vi "Autonomous Independent.vi"() -> ()   [LabVIEW 2016]
doc: "This VI is called when autonomous begins, and will automatically be terminated when autonomous ends. You can carry out timed or sensor driven robot movement independently without needing to return to the caller."
uses:
  Control Files/DriveMotors.ctl
  Control Files/SwerveMotors.ctl
panel:
  in  "error in":errorcluster
  # "Be sure to right-click and choose Data Operations>>Make Current Value default if you want to save the array values with the VI"
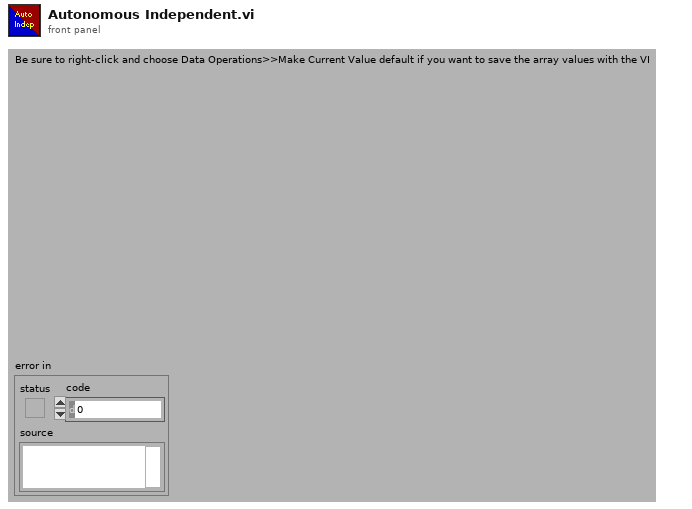
[diagram p1: front panel]
types:
  T1 = typedef "SwerveMotors.ctl" = enum16{"Swerve 1", "Swerve 2", "Swerve 3", "Swerve 4"}
  T2 = typedef "DriveMotors.ctl" = enum16{"Drive1", "Drive2", "Drive3", "Drive4"}
  T3 = typedef "WPI_MotorControlDeviceRef.ctl" = cluster{"DeviceStatus":errorcluster, "Type":T4, "PWM":cluster{"PWM Channel":T5, "DeadBand":T6}, "CAN":cluster{"Device Number":u8, "SetOutput VI Ref":variant, "GetOutput VI Ref":variant, "Enable VI Ref":variant, "Disable VI Ref":variant, "Data":variant}, "Invert":bool}
  T4 = typedef "WPI_MotorControlType.ctl" = enum16{"PWM", "CAN"}
  T5 = typedef "FPGA_DIOPWMChannel.ctl" = enum8{"PWM 0", "PWM 1", "PWM 2", "PWM 3", "PWM 4", "PWM 5", "PWM 6", "PWM 7", "PWM 8", "PWM 9", "PWM MXP 0", "PWM MXP 1", "PWM MXP 2", "PWM MXP 3", "PWM MXP 4", "PWM MXP 5", "PWM MXP 6", "PWM MXP 7", "PWM MXP 8", "PWM MXP 9", "Invalid"}
  T6 = typedef "WPI_PWMDeadband.ctl" = cluster{"Name":string, "maxPositivePwm":i32, "minPositivePwm":i32, "centerPwm":i32, "maxNegativePwm":i32, "minNegativePwm":i32, "angularRange":u16}
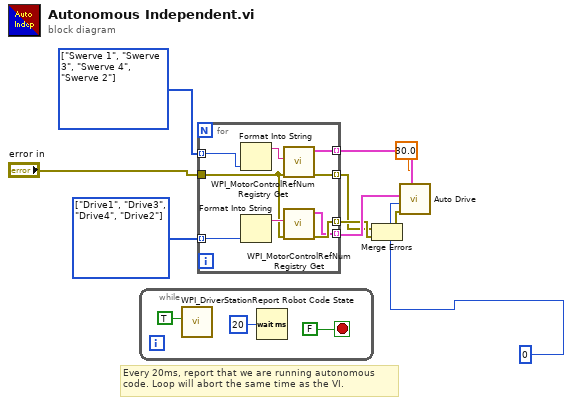
[diagram p0: block diagram]
diagram:
  w10 = T1[] [enum."Swerve 1", enum."Swerve 3", enum."Swerve 4", enum."Swerve 2"] items=["Swerve 1", "Swerve 2", "Swerve 3", "Swerve 4"] ("Array")
  w9 = T2[] [enum."Drive1", enum."Drive3", enum."Drive4", enum."Drive2"] items=["Drive1", "Drive2", "Drive3", "Drive4"] ("Array")
  # "Every 20ms, report that we are running autonomous\ncode. Loop will abort the same time as the VI."
  n1 = while {
    stop <- FALSE stop-if-true
    n2 = call <vilib>:"WPI_DriverStationReport Robot Code State.vi"("Autonomous"=TRUE) -> ()  [unwired: 10 in, 1 out]
    n3 = Wait (ms)(milliseconds to wait=u32 20) -> ()  [unwired: 1 out]
  }
  n4 = for {
    tunnel: w9 -> [w22] mode=indexing
    tunnel: w10 -> [w21] mode=indexing
    tunnel: "error in" -> [w18]
    tunnel: [w17] -> w5 mode=indexing
    tunnel: [w16] -> w3 mode=indexing
    tunnel: [w15] -> w7 mode=indexing
    tunnel: [w14] -> w6 mode=indexing
    n5 = Format Into String(w21) -> (resulting string=w20:string)  [unwired: 3 in, 1 out]
    n6 = Format Into String(w22) -> (resulting string=w19:string)  [unwired: 3 in, 1 out]
    n7 = call <vilib>:"WPI_MotorControlRefNum Registry Get.vi"("error in (no error)"=w18, "refnum name"=w20) -> ("error out"=w16:errorcluster, "MotorControlDevRef"=w15:T3)  [unwired: 8 in]
    n8 = call <vilib>:"WPI_MotorControlRefNum Registry Get.vi"("error in (no error)"=w18, "refnum name"=w19) -> ("error out"=w17:errorcluster, "MotorControlDevRef"=w14:T3)  [unwired: 8 in]
  }
  n9 = Merge Errors(w3, w5) -> (w4:errorcluster)
  n10 = call "Auto Drive.vi"("Distance"=30.0, "error in (no error)"=w4, "Angle"=0, "Drive"=w6, "Swerve"=w7) -> ()  [unwired: 6 in, 1 out]
